vi "testGenerateOverriddenSystemDefinition.vi"(8 "error in (no error)":errorcluster, 11 "TestCase in":refnum<class "VeriStandTestUtilitiesTests.lvclass">) -> (0 "error out":errorcluster, 3 "TestCase out":refnum<class "VeriStandTestUtilitiesTests.lvclass">)   [LabVIEW 2016, in "VeriStandTestUtilitiesTests.lvclass"]
uses:
  VeriStandTestUtilitiesTests.lvclass
  ConfigPropertyItem.ctl
  NationalInstruments.VeriStand.SystemDefinitionAPI
  <userlib>/_OpenG.lib/file/file.llb/Build Path - File Names Array - path__ogtk.vi
  <userlib>/_OpenG.lib/file/file.llb/Build Path - Traditional - path__ogtk.vi
  GetSystemDefinitionPropertyValue/GetSystemDefinitionPropertyValue_String.vi
  GetSystemDefinitionPropertyValue/GetSystemDefinitionPropertyValue_Bool.vi
  <vilib>/addons/_JKI Toolkits/VI Tester/TestCase.llb/TestCase.lvclass
  VeriStandTestUtilities.lvlib
  C:/Program Files (x86)/National Instruments/LabVIEW 2016/vi.lib/addons/_JKI Toolkits/VI Tester/TestCase.llb/TestCase.lvclass
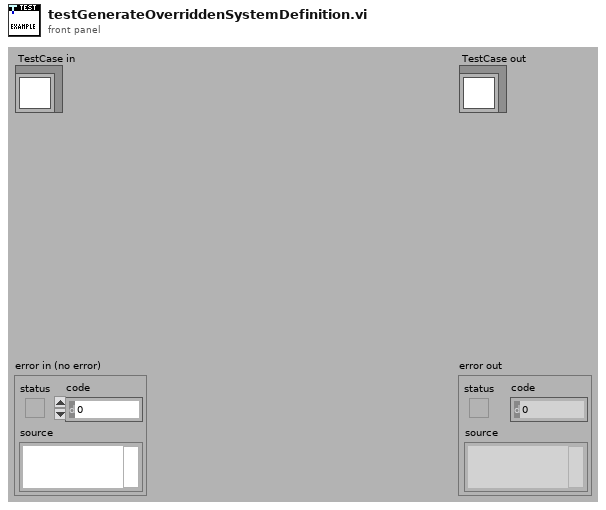
[diagram p1: front panel]
types:
  T1 = typedef "VeriStandTestUtilities.lvlib/ConfigPropertyItem.ctl" = cluster{"key":string, "value":string}
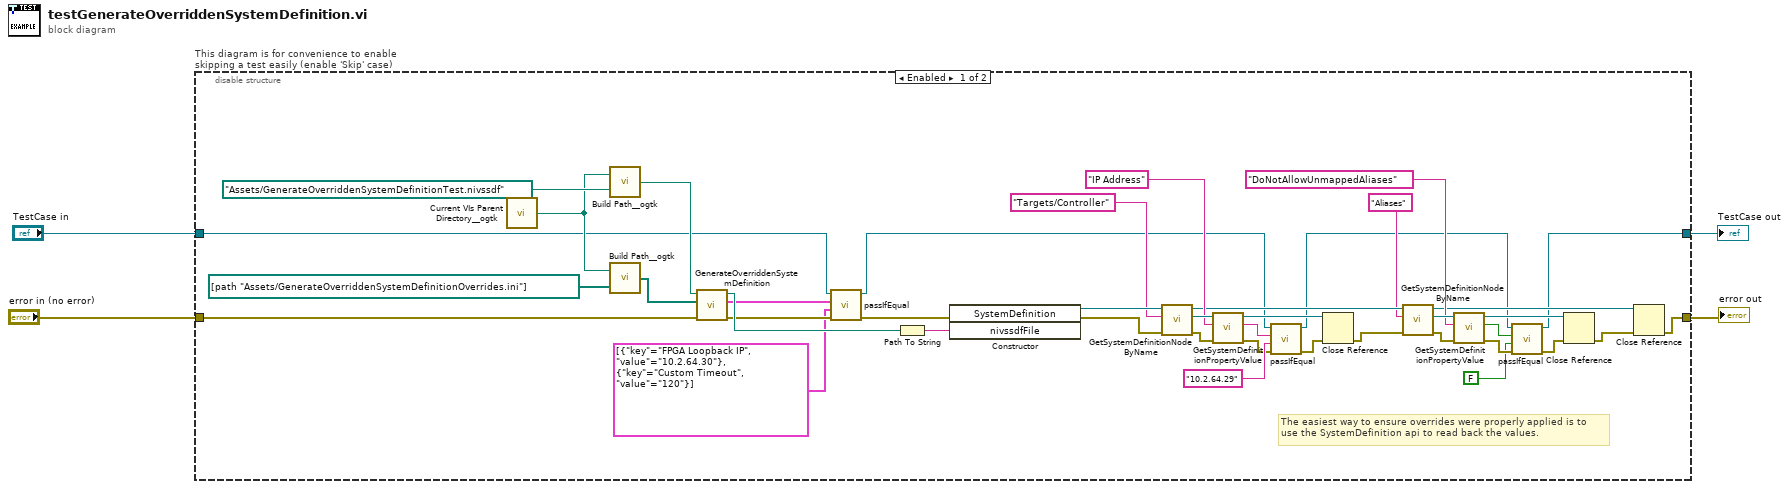
[diagram p0: block diagram]
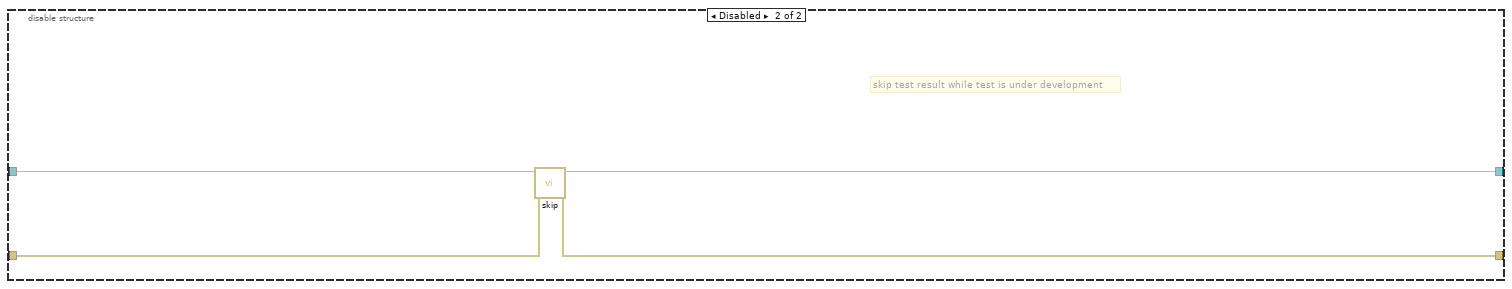
[diagram p2: hidden frame]
diagram:
  n1 = disable-structure "This diagram is for convenience to enable skipping a test easily (enable 'Skip' case)" shown="Enabled" {
    disable-tunnel: "TestCase in" -> [w8 w49]
    disable-tunnel: [w12 w47] -> w1
    disable-tunnel: [w26 w48] -> w3
    disable-tunnel: "error in (no error)" -> [w45 w46]
    frame Enabled {
      # "The easiest way to ensure overrides were properly applied is to\nuse the SystemDefinition api to read back the values."
      n2 = call <userlib>:"Current VIs Parent Directory__ogtk.vi"() -> ("Parent Directory (+ Relative)"=w31:path)  [unwired: 5 in]
      n3 = call-poly <userlib>:"Build Path__ogtk.vi"("name or relative path"=path "Assets/GenerateOverriddenSystemDefinitionTest.nivssdf" ("absolute system definition file"), "base path"=w31) -> ("appended path"=w32:path)
      n4 = call-poly <userlib>:"Build Path__ogtk.vi"("name or relative path"=path[] [path "Assets/GenerateOverriddenSystemDefinitionOverrides.ini"] ("absolute configuration files"), "base path"=w31) -> ("appended path"=w29:path[])
      n5 = call "GenerateOverriddenSystemDefinition.vi"("error in (no error)"=w45, "absolute configuration files"=w29, "absolute system definition file"=w32) -> ("error out"=w10:errorcluster, "properties"=w6:T1[], "absolute overridden system definition file"=w41:path)  [unwired: 5 in, 1 out]
      n6 = call-dynamic "passIfEqual.vi"("error in (no error)"=w10, "y"=T1[] [{"key"="FPGA Loopback IP", "value"="10.2.64.30"}, {"key"="Custom Timeout", "value"="120"}] ("properties"), "x"=w6, "TestCase in"=w8) -> ("error out"=w9:errorcluster, "TestCase out"=w7:refnum<class "VeriStandTestUtilitiesTests.lvclass">)  [unwired: 6 in]
      n7 = Path To String(path=w41) -> (string=w40:string)
      n8 = constructor class="SystemDefinition"(error in=w9, "nivssdfFile"=w40) -> (reference out=w39:refnum<k24>, error out=w42:errorcluster)  [unwired: 2 in, 2 out]
      n9 = call "GetSystemDefinitionNodeByName.vi"("error in (no error)"=w42, "nodepath"="Targets/Controller", "SystemDefinition in"=w39) -> ("error out"=w43:errorcluster, "BaseNodeType"=w44:refnum<k24>, "SystemDefinition out"=w18:refnum<k24>)  [unwired: 6 in]
      n10 = call-poly "GetSystemDefinitionPropertyValue.vi"("error in (no error)"=w43, "property name"="IP Address", "BaseNodeType in"=w44) -> ("error out"=w28:errorcluster, "value"=w35:string, "BaseNodeType out"=w27:refnum<k24>)  [unwired: 6 in]
      n11 = call-dynamic "passIfEqual.vi"("error in (no error)"=w28, "y"="10.2.64.29" ("property name"), "x"=w35, "TestCase in"=w7) -> ("error out"=w36:errorcluster, "TestCase out"=w13:refnum<class "VeriStandTestUtilitiesTests.lvclass">)  [unwired: 6 in]
      n12 = Close Reference(reference=w27, error in (no error)=w36) -> (error out=w17:errorcluster)
      n13 = call "GetSystemDefinitionNodeByName.vi"("error in (no error)"=w17, "nodepath"="Aliases", "SystemDefinition in"=w18) -> ("error out"=w24:errorcluster, "BaseNodeType"=w25:refnum<k24>, "SystemDefinition out"=w15:refnum<k24>)  [unwired: 6 in]
      n14 = call-poly "GetSystemDefinitionPropertyValue.vi"("error in (no error)"=w24, "property name"="DoNotAllowUnmappedAliases", "BaseNodeType in"=w25) -> ("error out"=w20:errorcluster, "value"=w21:bool, "BaseNodeType out"=w19:refnum<k24>)  [unwired: 6 in]
      n15 = call-dynamic "passIfEqual.vi"("error in (no error)"=w20, "y"=FALSE, "x"=w21, "TestCase in"=w13) -> ("error out"=w22:errorcluster, "TestCase out"=w12:refnum<class "VeriStandTestUtilitiesTests.lvclass">)  [unwired: 6 in]
      n16 = Close Reference(reference=w19, error in (no error)=w22) -> (error out=w14:errorcluster)
      n17 = Close Reference(reference=w15, error in (no error)=w14) -> (error out=w26:errorcluster)
    }
    frame Disabled {
      # "skip test result while test is under development"
      n18 = call <vilib>:"skip.vi"("error in (no error)"=w46, "TestCase in"=w49) -> ("error out"=w48:errorcluster, "TestCase out"=w47:refnum<class "VeriStandTestUtilitiesTests.lvclass">)  [unwired: 8 in]
    }
  }
  "error out" <- w3
  "TestCase out" <- w1
